vi "Get String.vi"(5 "use temporary file? (F)":bool, 7 "data type of variable":string, 8 "error in":errorcluster, 10 "variable name":string, 11 "GOLPI ref. in":T1={"pipe handle"={"lv_proc.dll file path"=path "", "process instance handle"=[], "debug mode"=FALSE, "debug data"=[]}, "fast read timeout [ms]"=500, "fast read settle time [ms]"=10, "fast read to multiple [ms]"=1, "max elements per input line"=100, "slow read timeout [ms]"=5000, "stdin double format specifier"="%_16e", "max elements per stdout output column"=100, "console mode bitstream"=FALSE, "bitstream first read timeout [ms]"=1000, "bitstream read timeout [ms]"=50, "struct transfer possible"=FALSE}) -> (0 "error out":errorcluster, 2 "value":string, 3 "GOLPI ref. out":T1={"pipe handle"={"lv_proc.dll file path"=path "", "process instance handle"=[], "debug mode"=FALSE, "debug data"=[]}, "fast read timeout [ms]"=500, "fast read settle time [ms]"=10, "fast read to multiple [ms]"=1, "max elements per input line"=100, "slow read timeout [ms]"=5000, "stdin double format specifier"="%_16e", "max elements per stdout output column"=100, "console mode bitstream"=FALSE, "bitstream first read timeout [ms]"=1000, "bitstream read timeout [ms]"=50, "struct transfer possible"=FALSE})   [LabVIEW 2013, in "GOLPI library.lvlib"]
doc: "Part of polymorph Get Variable.vi"
uses:
  GOLPI library.lvlib
  Public/GOLPI reference Type Def.ctl
  LV Process source distribution/Pipe Handle.ctl
  Type Definitions/Bitstream Data Type.ctl
  Type Definitions/Custom Error Codes Enum Type Def.vi
  LV Process source distribution/LV Process library.lvlib
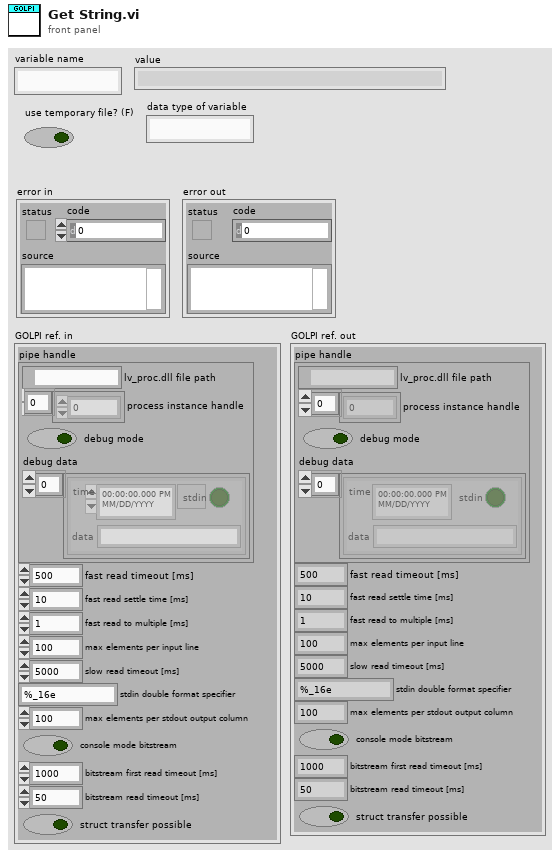
[diagram p1: front panel]
types:
  T1 = typedef "GOLPI library.lvlib/GOLPI reference Type Def.ctl" = cluster{"pipe handle":T2, "fast read timeout [ms]":u32, "fast read settle time [ms]":u32, "fast read to multiple [ms]":u32, "max elements per input line":u32, "slow read timeout [ms]":u32, "stdin double format specifier":string, "max elements per stdout output column":u32, "console mode bitstream":bool, "bitstream first read timeout [ms]":u32, "bitstream read timeout [ms]":u32, "struct transfer possible":bool}
  T2 = typedef "LV Process library.lvlib/Pipe Handle.ctl" = cluster{"lv_proc.dll file path":path, "process instance handle":u32[], "debug mode":bool, "debug data":cluster{"time":timestamp, "stdin":bool, "data":string}[]}
  T3 = typedef "GOLPI library.lvlib/Bitstream Data Type.ctl" = enum16{"dummy", "int", "uint", "float", "complex", "str", "real numeric"}
  T4 = typedef "GOLPI library.lvlib/Custom Error Codes Enum Type Def.vi" = enum16{"no error", "00 working directory PAR1 missing", "01 octave binary PAR1 missing", "02 octave report error PAR1", "03 empty output last cmd PAR1", "04 missing temporary file PAR1", "05 pwd PAR 1 not exist", "10 var PAR1 not string, vect", "11 var PAR1 not num, scal, ~compl", "12 var PAR1 not num, scal, compl", "13 var PAR1 not num, vect, ~compl", "14 var PAR1 not num, vect, compl", "15 var PAR1 not num, mat, ~compl", "16 var PAR1 not num, mat, ~compl", "30 read timeout", "60 bitstream transport failed", "61 bitstream decode error PAR1", "62 bitstream cannot be set", "70 struct transfer not possible", "80 struct: cluster elem. PAR1 not implem.", "81 struct: structure field PAR1 not implem.", "82 struct: size mismatch of PAR1", "83 struct: type mismatch of PAR1", "98 internal error", "99 not finished"}
  T5 = typedef "GOLPI library.lvlib/Bitstream Data.ctl" = cluster{"double":dbl[][], "cplx double":cdb[][], "int64":i64[][], "uint64":u64[][], "str":string[], "data type":T3}
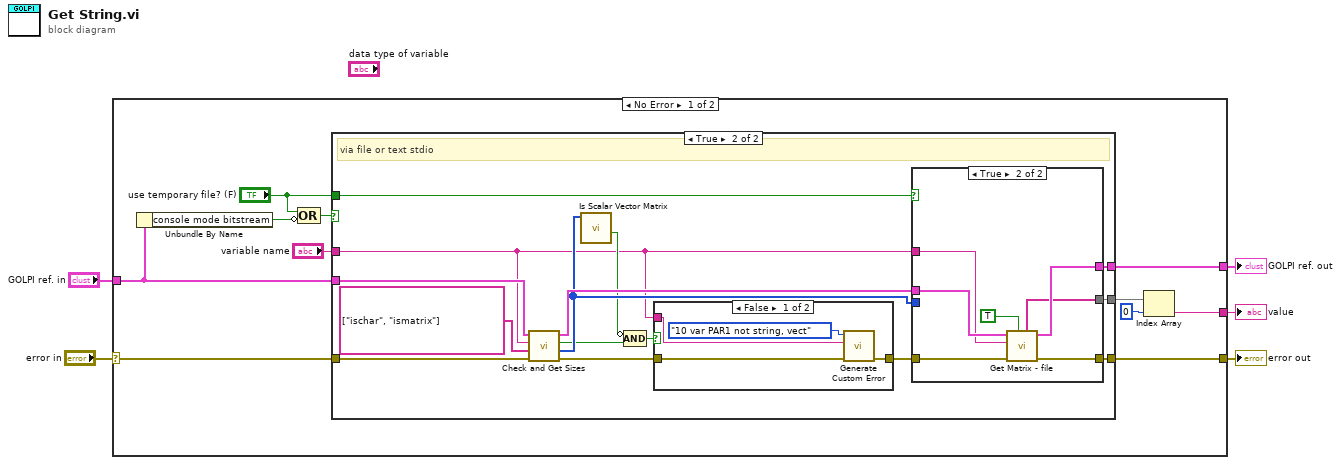
[diagram p0: block diagram]
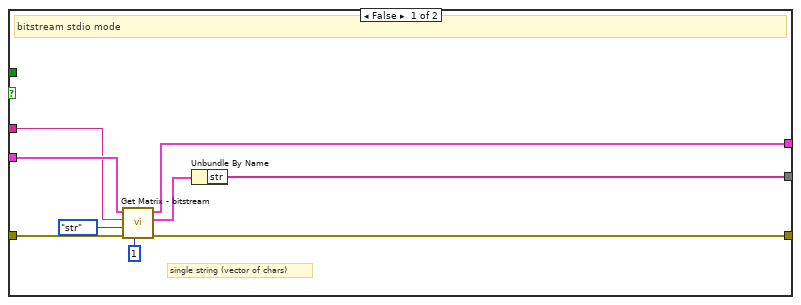
[diagram p2: hidden frame]
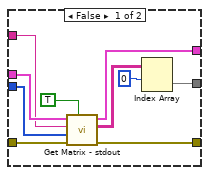
[diagram p3: hidden frame]
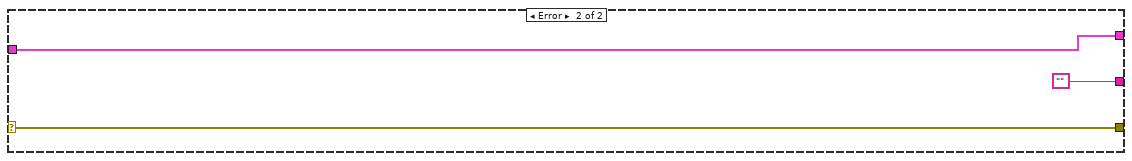
[diagram p5: hidden frame]
diagram:
  n1 = case shown="No Error" "error in" {
    selector: "error in" -> [w16 w64]
    tunnel: [w12 w64] -> w5
    tunnel: [w11 ""] -> w4
    tunnel: "GOLPI ref. in" -> [w10 w63]
    tunnel: [w15 w63] -> w1
    frame No Error {
      n2 = Unbundle By Name(w10) -> ("console mode bitstream"=w9:bool)
      n3 = Compound Arithmetic op=OR("use temporary file? (F)", invert w9) -> (w7:bool)
      n4 = case shown="True" w7 {
        tunnel: w16 -> [w25 w39]
        tunnel: w10 -> [w24 w37]
        tunnel: [w20 w34] -> w15
        tunnel: [w18 w33] -> w13
        tunnel: [w17 w32] -> w12
        tunnel: "use temporary file? (F)" -> [_ w27]
        tunnel: "variable name" -> [w21 w26]
        frame False {
          # "single string (vector of chars)"
          # "bitstream stdio mode"
          n5 = call "Get Matrix - bitstream.vi"("max dimensions (0: scalar)"=1, "error in (no error)"=w25, "data type"=Bitstream_Data_Type."str", "variable name"=w21, "GOLPI ref. in"=w24) -> ("error out"=w17:errorcluster, "data"=w19:T5, "GOLPI ref. out"=w20:T1)  [unwired: 4 in]
          n6 = Unbundle By Name(w19) -> ("str"=w18:string[])
        }
        frame True {
          # "via file or text stdio"
          n7 = call "Check and Get Sizes.vi"("error in (no error)"=w39, "test commands"=string[] ["ischar", "ismatrix"], "variable name"=w26, "GOLPI ref. in"=w37) -> ("error out"=w40:errorcluster, "octave sizes"=w31:i32[], "all tests OK?"=w30:bool, "GOLPI ref. out"=w35:T1)  [unwired: 4 in]
          n8 = call "Is Scalar Vector Matrix.vi"("octave sizes"=w31) -> ("is matrix?"=w28:bool)  [unwired: 5 in, 5 out]
          n9 = Compound Arithmetic op=AND(invert w28, w30) -> (w29:bool)
          n10 = case shown="False" w29 {
            tunnel: [w60 w62] -> w36
            tunnel: w40 -> [w61 w62]
            tunnel: w26 -> [w59 _]
            frame False {
              n11 = call "Generate Custom Error.vi"("error in"=w61, "PAR1"=w59, "GOLPI error"=Custom_Error_Codes_Enum_Type_Def.vi."10 var PAR1 not string, vect" ("Enum")) -> ("error out"=w60:errorcluster)  [unwired: 8 in]
            }
            frame True {
            }
          }
          n12 = case shown="True" w27 {
            tunnel: w36 -> [w50 w57]
            tunnel: [w49 w55] -> w32
            tunnel: w35 -> [w48 w56]
            tunnel: [w47 w54] -> w34
            tunnel: w26 -> [w45 w52]
            tunnel: w31 -> [w44 _]
            tunnel: [w41 w51] -> w33
            frame False {
              n13 = call "Get Matrix - stdout.vi"("is string?"=TRUE ("is string"), "error in (no error)"=w50, "octave sizes"=w44, "variable name"=w45, "GOLPI ref. in"=w48) -> ("error out"=w49:errorcluster, "array"=w42:string[][], "GOLPI ref. out"=w47:T1)  [unwired: 4 in]
              n14 = Index Array(array=w42, index (row)=0) -> (element=w41:string[])  [unwired: 1 in]
            }
            frame True {
              n15 = call "Get Matrix - file.vi"("is string?"=TRUE ("is string"), "error in (no error)"=w57, "variable name"=w52, "GOLPI ref. in"=w56) -> ("error out"=w55:errorcluster, "GOLPI ref. out"=w54:T1, "string array"=w51:string[])  [unwired: 3 in, 2 out]
            }
          }
        }
      }
      n16 = Index Array(array=w13, index=0 ("index (row)")) -> (element=w11:string)
    }
    frame Error {
    }
  }
  "value" <- w4
  "error out" <- w5
  "GOLPI ref. out" <- w1
